vi "OSQ_load.vi"(8 "error in (no error)":errorcluster, 11 "Open":path=path "C:/Users/Adam/Desktop/test.osq") -> (0 "error out":errorcluster, 2 "SEQs":T1[](array[typedef]), 3 "XML File Path(duplicate)":path, 4 "Lines":i32)   [LabVIEW 2013]
uses:
  Line.ctl
  <vilib>/Utility/xml.llb/Read From XML File(string).vi
panel:
  out "XML Elements":string
  in  "Template":T1[](array[typedef])
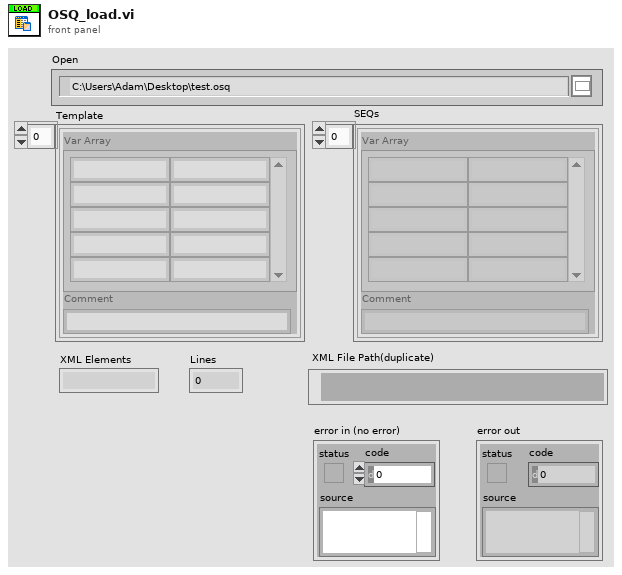
[diagram p1: front panel]
types:
  T1 = typedef "Line.ctl" = cluster{"Var Array":string[][], "Comment":string}
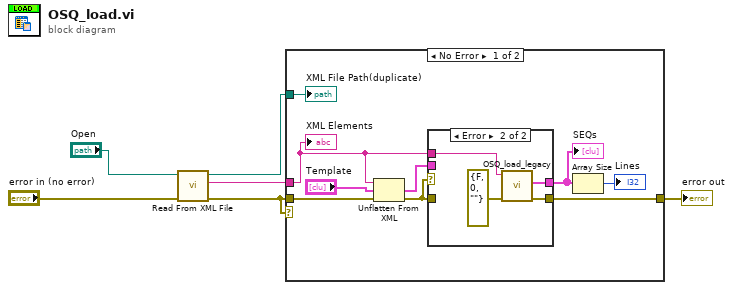
[diagram p0: block diagram]
diagram:
  n1 = call-poly <vilib>:"Read From XML File.vi"("error in (no error)"="error in (no error)", "XML File Path"="Open") -> ("error out"=w2:errorcluster, "XML Elements"=w3:string, "XML File Path(duplicate)"=w4:path)  [unwired: 7 in]
  n2 = case shown="No Error" w2 {
    tunnel: w4 -> [w15 _]
    tunnel: w3 -> [w11 _]
    tunnel: w2 -> [w13 w22]
    tunnel: [w9 w22] -> w1
    frame No Error {
      n3 = Unflatten From XML(xml string=w11, type="Template", error in (no error)=w13) -> (value=w12:T1[], error out=w10:errorcluster)
      n4 = case shown="Error" w10 {
        tunnel: w12 -> [w17 _]
        tunnel: [w17 w20] -> w8
        tunnel: w11 -> [_ w21]
        tunnel: w10 -> [w16 _]
        tunnel: [w16 w19] -> w9
        frame No Error {
        }
        frame Error {
          n5 = call "OSQ_load_legacy.vi"("error in (no error)"=errorcluster {"status"=FALSE, "code"=0, "source"=""}, "XML Elements"=w21) -> ("error out"=w19:errorcluster, "SEQs"=w20:T1[])  [unwired: 8 in]
        }
      }
      "SEQs" <- w8
      n6 = Array Size(array=w8) -> (size(s)=→"Lines":i32)
      "XML File Path(duplicate)" <- w15
      "XML Elements" <- w11
    }
    frame Error {
    }
  }
  "error out" <- w1
